vi "DEVICE MAIN.vi"() -> ()   [LabVIEW 2015]
uses:
  <vilib>/Espotel/IoT Foundation/IoTF/CTLs/IoTF Device Subscription.ctl
  <vilib>/Espotel/IoT Foundation/MQTT/Public CTLs/MQTT QoS.ctl
  <vilib>/Espotel/IoT Foundation/IoTF/CTLs/IoTF Device Credentials.ctl
  <vilib>/Espotel/IoT Foundation/IoTF/CTLs/IoTF Message.ctl
  <vilib>/myRIO/Common/Instrument Driver Framework/myRIO v1.0/UART/vis/myRIO v1.0 Close UART.vi
  <vilib>/myRIO/Common/Instrument Driver Framework/Utilities/vis/FPGA Ref Manager.vi
  <vilib>/myRIO/Common/Instrument Driver Framework/myRIO v1.0/myRIO v1.0 Reset FPGA.vi
  <vilib>/myRIO/Common/Instrument Driver Framework/myRIO v1.0/IRQ/vis/myRIO v1.0 IRQ Info FGV.vi
  <vilib>/myRIO/Common/Instrument Driver Framework/myRIO v1.0/IRQ/vis/myRIO v1.0 Timer IRQ Info FGV.vi
  <vilib>/myRIO/Common/Instrument Driver Framework/myRIO v1.0/IRQ/vis/myRIO v1.0 ISR Agent.vi
  <vilib>/Espotel/IoT Foundation/IoTF/IoTF Library.lvlib
  <vilib>/Espotel/IoT Foundation/MQTT/MQTT Library.lvlib
  <vilib>/myRIO/Instrument Drivers/Utilities/Utilities.lvlib
panel:
  out "Obstacle":bool
  out "Y":i8
  out "Yeah Magnets!!":bool
  out "Z":i8
  out "Flame":bool
  out "X":i8
  in  "Process Stop Button":bool
  out "Sound":sgl[](graph)
  # "Device"
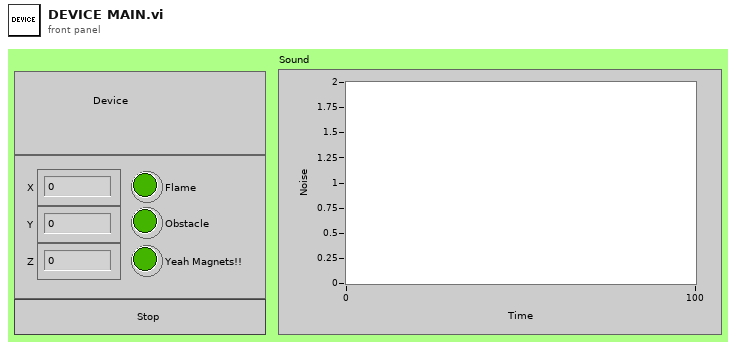
[diagram p1: front panel]
types:
  T1 = typedef "IoTF Library.lvlib/IoTF Device Credentials.ctl" = cluster{"Organization ID":string, "Device Type":string, "Device ID":string, "Auth-token":string}
  T2 = typedef "IoTF Library.lvlib/IoTF Device Subscription.ctl" = cluster{"Subscription":string, "QoS":T3}
  T3 = typedef "MQTT Library.lvlib/MQTT QoS.ctl" = enum16{"At most once", "At least once", "Exactly once"}
  T4 = typedef "IoTF Library.lvlib/IoTF Message.ctl" = cluster{"Message ID":string, "JSON object":string, "QoS":T3, "Include timestamp?":bool, "Custom JSON payload?":bool}
  T5 = typedef "Sensors Data.ctl" = cluster{"X":i8, "Y":i8, "Z":i8, "flame":bool, "magnet":bool, "obstacle":bool, "sound":sgl[]}
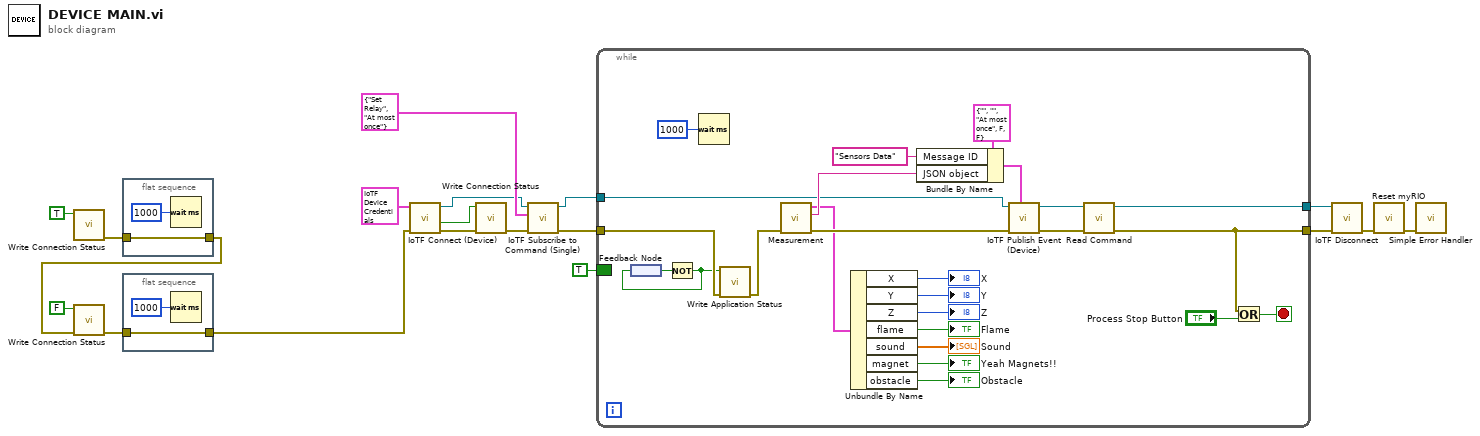
[diagram p0: block diagram]
diagram:
  n1 = call "Write Connection Status.vi"("status"=TRUE) -> ("error out"=w6:errorcluster)  [unwired: 10 in]
  n2 = call "Write Connection Status.vi"("error in (no error)"=w2, "status"=FALSE) -> ("error out"=w3:errorcluster)  [unwired: 9 in]
  n3 = flat-sequence {
    tunnel: w6 -> [w21]
    tunnel: [w21] -> w2
    frame #0 {
      n4 = Wait (ms)(milliseconds to wait=u32 1000) -> ()  [unwired: 1 out]
    }
  }
  n5 = flat-sequence {
    tunnel: w3 -> [w23]
    tunnel: [w23] -> w1
    frame #0 {
      n6 = Wait (ms)(milliseconds to wait=u32 1000) -> ()  [unwired: 1 out]
    }
  }
  n7 = call <vilib>:"IoTF Connect (Device).vi"("Error in (no error)"=w1, "IoTF Device Credentials"=T1 {"Organization ID"="hlkhwz", "Device Type"="LabVIEW_Minion", "Device ID"="Minion-00", "Auth-token"="V56OmlJPpDtL1BPfkK"}) -> ("Error out"=w9:errorcluster, "Connection accepted?"=w8:bool, "Connection ID out"=w12:refnum<k5>)  [unwired: 5 in, 2 out]
  n8 = call "Write Connection Status.vi"("error in (no error)"=w9, "status"=w8) -> ("error out"=w14:errorcluster)  [unwired: 9 in]
  n9 = call <vilib>:"IoTF Subscribe to Command (Single).vi"("Error in (no error)"=w14, "Subscription"=T2 {"Subscription"="Set Relay", "QoS"=enum."At most once"}, "Connection ID in"=w12) -> ("Error out"=w18:errorcluster, "Connection ID out"=w17:refnum<k5>)  [unwired: 5 in, 2 out]
  n10 = while {
    tunnel: w18 -> [w47]
    tunnel: [w36] -> w16
    border: TRUE -> [_]
    tunnel: w17 -> [w37]
    tunnel: [w35] -> w7
    stop <- w45 stop-if-true
    n11 = feedback #1() -> (w44:bool)
    n12 = Not(x=w44) -> (.not. x?=w43:bool)
    n13 = feedback-in #1(w43) -> ()
    n14 = Wait (ms)(milliseconds to wait=u32 1000) -> ()  [unwired: 1 out]
    n15 = call "Write Application Status.vi"("error in (no error)"=w47, "status"=w43) -> ("error out"=w46:errorcluster)  [unwired: 9 in]
    n16 = call "Measurement.vi"("error in (no error)"=w46) -> ("error out"=w40:errorcluster, "JSON object"=w39:string, "sensors data"=w33:T5)  [unwired: 8 in]
    n17 = Unbundle By Name(w33) -> ("X"=→"X":i8, "Y"=→"Y":i8, "Z"=→"Z":i8, "flame"=→"Flame":bool, "sound"=→"Sound":sgl[], "magnet"=→"Yeah Magnets!!":bool, "obstacle"=→"Obstacle":bool)
    n18 = Bundle By Name(cluster=T4 {"Message ID"="", "JSON object"="", "QoS"=enum."At most once", "Include timestamp?"=FALSE, "Custom JSON payload?"=FALSE} ("IoTF Message"), "Message ID"="Sensors Data", "JSON object"=w39) -> (w38:T4)
    n19 = call <vilib>:"IoTF Publish Event (Device).vi"("IoTF Message"=w38, "Error in (no error)"=w40, "Connection ID in"=w37) -> ("Error out"=w27:errorcluster, "Connection ID out"=w24:refnum<k5>)  [unwired: 6 in, 1 out]
    n20 = call "Read Command.vi"("error in (no error)"=w27, "Connection ID in"=w24) -> ("error out"=w36:errorcluster, "Connection ID out"=w35:refnum<k5>)  [unwired: 8 in]
    n21 = Or(x=w36, y="Process Stop Button") -> (x .or. y?=w45:bool)
  }
  n22 = call <vilib>:"IoTF Disconnect.vi"("Error in (no error)"=w16, "Connection ID in"=w7) -> ("Error out"=w15:errorcluster)  [unwired: 8 in, 1 out]
  n23 = call <vilib>:"Reset myRIO.vi"("error in (no error)"=w15) -> ("error out"=w19:errorcluster)  [unwired: 10 in]
  n24 = call <vilib>:"Simple Error Handler.vi"("error in (no error)"=w19) -> ()  [unwired: 4 in, 5 out]
